vi "Hello World.vi"   [LabVIEW 2018]
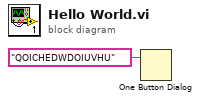
[diagram p0: block diagram]
diagram:
  n1 = One Button Dialog(message="QOICHEDWDOIUVHU") -> ()  [unwired: 1 in, 1 out]
